vi "UI Panels - Set Panel Properties.vi"(4 "Collapsable (T)":bool=TRUE, 5 "Expanded by Default (T)":bool=TRUE, 6 "Resizible (T)":bool=TRUE, 7 "index":i32, 8 "error in (no error)":errorcluster, 10 "Height":cluster{"Collapsed":i32, "Expanded":i32}={"Collapsed"=100, "Expanded"=250}, 11 "Panels_XControl":refnum<vi>) -> (0 "error out":errorcluster, 3 "Panels_XControl Out":refnum<vi>)   [LabVIEW 2013, in "UI Panels.lvlib"]
uses:
  UI Panels.lvlib
  Panels_XControl.xctl
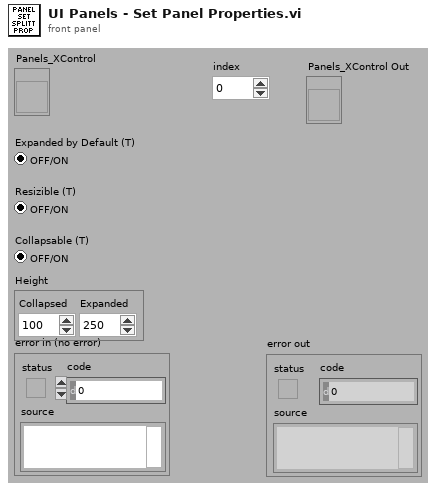
[diagram p1: front panel]
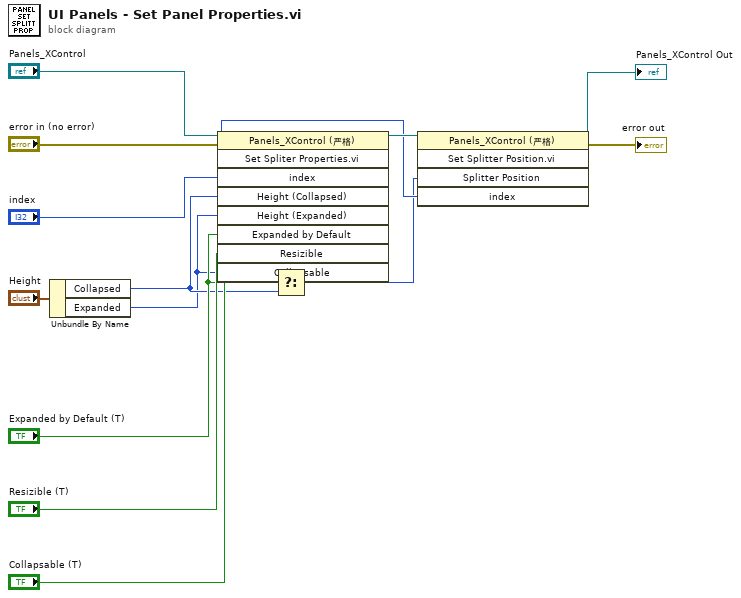
[diagram p0: block diagram]
diagram:
  n1 = Unbundle By Name("Height") -> ("Collapsed"=w2:i32, "Expanded"=w1:i32)
  n2 = invoke on="Invoke Node" class="Panels_XControl (严格)" method="Set Spliter Properties.vi"(reference="Panels_XControl", error in="error in (no error)", "index"="index", "Height (Collapsed)"=w2, "Height (Expanded)"=w1, "Expanded by Default"="Expanded by Default (T)", "Resizible"="Resizible (T)", "Collapsable"="Collapsable (T)") -> (reference out=w9:refnum<vi>)  [unwired: 1 in, 8 out]
  n3 = Select(t=w1, s="Expanded by Default (T)", f=w2) -> (s? t:f=w6:i32)
  n4 = invoke on="Invoke Node" class="Panels_XControl (严格)" method="Set Splitter Position.vi"(reference=w9, "Splitter Position"=w6, "index"="index") -> (reference out=→"Panels_XControl Out":refnum<vi>, error out=→"error out":errorcluster)  [unwired: 2 in, 3 out]
